vi "Add Key Value To Profile.vi"(9 "Value":string, 10 "Key":string, 11 "Descriptor":string) -> (3 "Flavoured Descriptor":string)   [LabVIEW 2015]
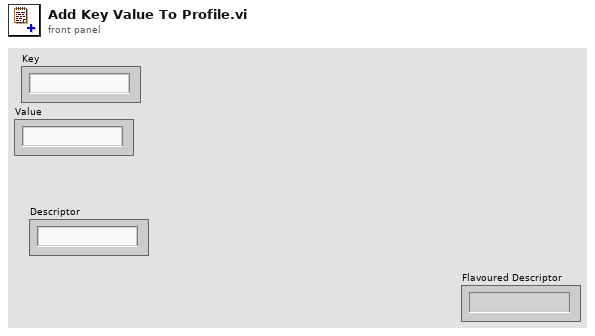
[diagram p1: front panel]
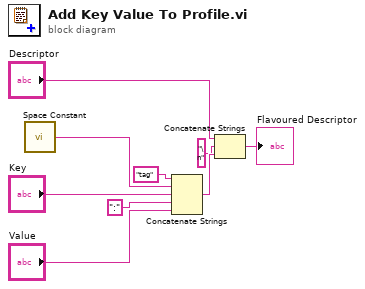
[diagram p0: block diagram]
diagram:
  n1 = call <vilib>:"Space Constant.vi"() -> ("String"=w4:string)
  n2 = Concatenate Strings("tag", w4, "Key", ":" ("string"), "Value") -> (w6:string)
  n3 = Concatenate Strings("Descriptor", "\n" ("string"), w6) -> (→"Flavoured Descriptor":string)
